vi "Activate.vi"(8 "error in (no error)":errorcluster, 11 "Object ref in":T1) -> (0 "error out":errorcluster, 3 "Object ref out":T1)   [LabVIEW 2013, in "SLMControl.lvlib" / "SC-Main.lvclass"]
uses:
  SC-Main.lvclass
  Object-reference.ctl
  SC-Main.lvclass/SC-Main.ctl
  Application-status.ctl
  Lasing-actions.ctl
  UI/Control-names.ctl
  Deposition-actions.ctl
  Read UI.vi
  Read Status.vi
  UI/Set-control-enable-multiple.vi
  UI/Set-control-enable-single.vi
  UI/Set-control-boolean.vi
  UI/SC-UI.lvclass
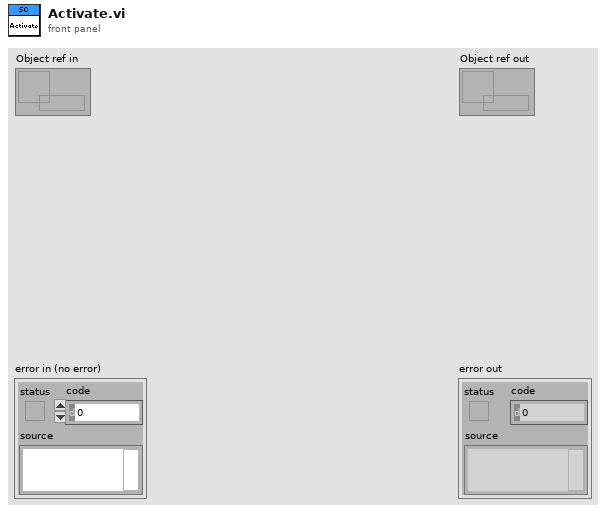
[diagram p1: front panel]
types:
  T1 = typedef "SLMControl.lvlib/SC-Main.lvclass/Object-reference.ctl" = refnum<data-value>
  T2 = typedef "SLMControl.lvlib/SC-UI.lvclass/Control-names.ctl" = enum16{"Com-in", "Com-out", "Help", "Status", "Load configuration", "Save configuration", "Load lasing files", "Load deposition files", "Clear", "Files", "Activate", "Execute", "Abort", "Options", "Current layer", "Current iteration", "Last elapsed time", "Deposition status", "Lasing job", "Status LEDs", "Exiting led", "Initialized led", "Files loaded led", "Activated led", "Executing led", "Deposition led", "Lasing job led", "Lasing led"}
  T3 = typedef "SLMControl.lvlib/SC-Main.lvclass/Lasing-actions.ctl" = enum16{"Idle", "Activate", "Load lasing file", "Launch lasing", "Wait for lasing end", "Signal iterate", "Signal abort", "Abort", "Reset", "Exit"}
  T4 = typedef "SLMControl.lvlib/SC-Main.lvclass/Application-status.ctl" = enum16{"Idle", "Initialized", "Configured", "Activated", "Started", "Paused", "Stopped", "Reset", "Error", "Exited"}
  T5 = typedef "SLMControl.lvlib/SC-Main.lvclass/Deposition-actions.ctl" = enum16{"Idle", "Activate", "Load deposition", "Launch deposition", "Wait for deposition end", "Signal lasing", "Abort", "Reset", "Exit"}
  T6 = typedef "SLMControl.lvlib/SC-Main.lvclass/Client-status.ctl" = enum16{"Idle", "Initialized", "Configured", "Activated", "Started", "Paused", "Stopped", "Reset", "Error", "Exited"}
  T7 = typedef "SLMControl.lvlib/SC-UI.lvclass/Panes-reference.ctl" = refnum<data-value>
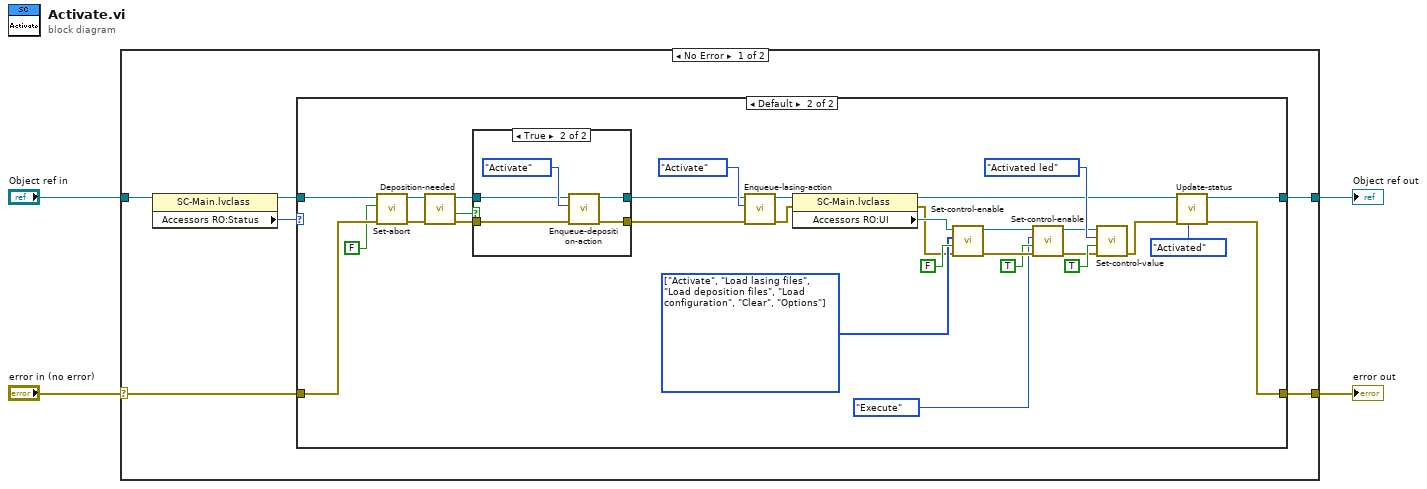
[diagram p0: block diagram]
diagram:
  n1 = case shown="No Error" "error in (no error)" {
    selector: "error in (no error)" -> [w7 w51]
    tunnel: [w10 w51] -> w3
    tunnel: [w9 w50] -> w1
    tunnel: "Object ref in" -> [w8 w50]
    frame No Error {
      n2 = property class="SC-Main.lvclass"(reference=w8) -> (reference out=w6:T1, "Accessors RO:Status"=w5:T6)  [unwired: 1 in, 1 out]
      n3 = case shown="Default" w5 {
        tunnel: [w11 w41] -> w10
        tunnel: [w12 w40] -> w9
        tunnel: w7 -> [w11 w24]
        tunnel: w6 -> [w12 w21]
        frame "Initialized", "Started", "Paused" {
        }
        frame Default {
          w31 = T2[] [enum."Activate", enum."Load lasing files", enum."Load deposition files", enum."Load configuration", enum."Clear", enum."Options"] items=["Com-in", "Com-out", "Help", "Status", "Load configuration", "Save configuration", "Load lasing files", "Load deposition files", "Clear", "Files", "Activate", "Execute", "Abort", "Options", "Current layer", "Current iteration", "Last elapsed time", "Deposition status", "Lasing job", "Status LEDs", "Exiting led", "Initialized led", "Files loaded led", "Activated led", "Executing led", "Deposition led", "Lasing job led", "Lasing led"] ("Control names")
          n4 = call "Set-abort.vi"("error in (no error)"=w24, "Abort"=FALSE, "Object ref in"=w21) -> ("error out"=w18:errorcluster, "Object ref out"=w19:T1)  [unwired: 7 in]
          n5 = call "Deposition-needed.vi"("error in (no error)"=w18, "Object ref in"=w19) -> ("error out"=w16:errorcluster, "Deposit?"=w17:bool, "Object ref out"=w15:T1)  [unwired: 7 in]
          n6 = case shown="True" w17 {
            tunnel: [w44 w48] -> w14
            tunnel: [w43 w47] -> w13
            tunnel: w16 -> [w43 w46]
            tunnel: w15 -> [w44 w45]
            frame False {
            }
            frame True {
              n7 = call "Enqueue-deposition-action.vi"("error in (no error)"=w46, "Action"=Deposition-actions."Activate" ("Execution action"), "State queue in"=w45) -> ("error out"=w47:errorcluster, "State queue out"=w48:T1)  [unwired: 6 in, 1 out]
            }
          }
          n8 = call "Enqueue-lasing-action.vi"("error in (no error)"=w13, "Action"=Lasing-actions."Activate" ("Execution action"), "State queue in"=w14) -> ("error out"=w35:errorcluster, "State queue out"=w38:T1)  [unwired: 6 in, 1 out]
          n9 = property class="SC-Main.lvclass"(reference=w38, error in=w35) -> (reference out=w36:T1, error out=w30:errorcluster, "Accessors RO:UI"=w32:T7)
          n10 = call-poly "Set-control-enable.vi"("error in (no error)"=w30, "Enable?"=FALSE, "Control names"=w31, "Panes in"=w32) -> ("error out"=w28:errorcluster, "Panes out"=w29:T7)  [unwired: 6 in]
          n11 = call-poly "Set-control-enable.vi"("error in (no error)"=w28, "Enable?"=TRUE, "Control name"=Control-names."Execute", "Panes in"=w29) -> ("error out"=w25:errorcluster, "Panes out"=w26:T7)  [unwired: 6 in]
          n12 = call-poly "Set-control-value.vi"("error in (no error)"=w25, "Value"=TRUE, "Control name"=Control-names."Activated led", "Panes in"=w26) -> ("error out"=w20:errorcluster)  [unwired: 6 in, 1 out]
          n13 = call "Update-status.vi"("Status"=Application-status."Activated", "error in (no error)"=w20, "Object ref in"=w36) -> ("error out"=w41:errorcluster, "Object ref out"=w40:T1)  [unwired: 7 in]
        }
      }
    }
    frame Error {
    }
  }
  "error out" <- w3
  "Object ref out" <- w1
